vi "niRFUtil MASMT Util Error Out From Error Code.vi"(8 "error in (no error)":errorcluster, 11 "error code":i32) -> (0 "error out":errorcluster)   [LabVIEW 2016, in "niRFUtil.lvlib"]
uses:
  niRFUtil.lvlib
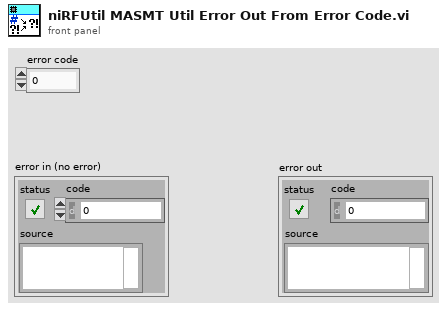
[diagram p1: front panel]
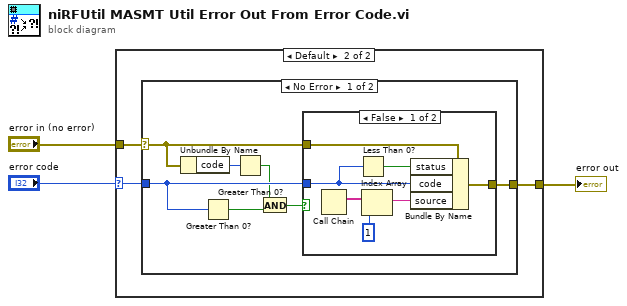
[diagram p0: block diagram]
diagram:
  n1 = case shown="Default" "error code" {
    selector: "error code" -> [_ w5]
    tunnel: "error in (no error)" -> [w4 w7]
    tunnel: [w4 w6] -> w1
    frame 0 {
    }
    frame Default {
      n2 = case shown="No Error" w7 {
        selector: w7 -> [w13 w23]
        tunnel: [w14 w23] -> w6
        tunnel: w5 -> [w12 _]
        frame No Error {
          n3 = Unbundle By Name(w13) -> ("code"=w11:i32)
          n4 = Greater Than 0?(x=w12) -> (x > 0?=w9:bool)
          n5 = Greater Than 0?(x=w11) -> (x > 0?=w10:bool)
          n6 = And(x=w10, y=w9) -> (x .and. y?=w8:bool)
          n7 = case shown="False" w8 {
            tunnel: w12 -> [w15 _]
            tunnel: [w20 w22] -> w14
            tunnel: w13 -> [w21 w22]
            frame False {
              n8 = Call Chain() -> (call chain=w19:string[])
              n9 = Less Than 0?(x=w15) -> (x < 0?=w16:bool)
              n10 = Index Array(array=w19, index=1) -> (element=w17:string)
              n11 = Bundle By Name(cluster=w21, "status"=w16, "code"=w15, "source"=w17) -> (w20:errorcluster)
            }
            frame True {
            }
          }
        }
        frame Error {
        }
      }
    }
  }
  "error out" <- w1
